vi "1DTurnMain.vi"() -> ()   [LabVIEW 2017]
panel:
  in  "StartAngle":dbl
  out "Done?":bool
  out "Vel":cluster{"Output":dbl, "dx/dt":dbl}(graph)={"Output"=0.0, "dx/dt"=-2.5707427177340247}
  in  "Gains":T1={"FFV"=0.0021, "FFA"=0.0001, "Vel PID"={"P"=0.002, "I"=0.0, "D"=0.0}} {"Vel PID"."D" format="%.3f"; "Vel PID"."I" format="%.3f"; "Vel PID"."P" format="%.3f"}
  out "Pos":dbl(graph)=90.04058722264358
  in  "Config":T2={"Gear Reduction"=15.0, "Wheel Radius (m)"=0.076, "# Motors"=6, "coeff of friction"=0.1, "Mass (kg)"=50.0, "Motor"={"Ke (V)"=0.0183, "R (ohms)"=0.09, "KT (Nm/A)"=0.0183, "Tf (Nm)"=0.4}}
  in  "TargetAngle":dbl=90.0
  in  "MaxVel":dbl=300.0
  in  "MaxAccel":dbl=400.0
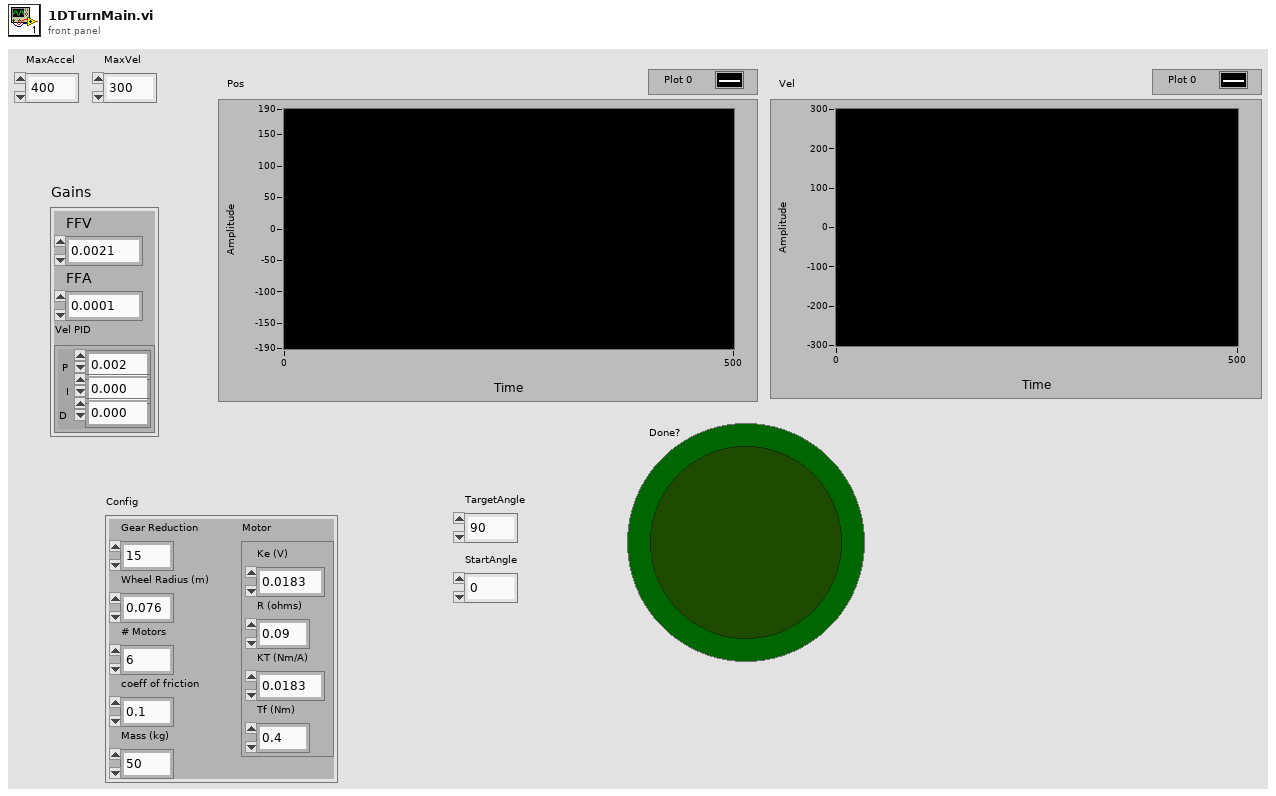
[diagram p1: front panel]
types:
  T1 = cluster{"FFV":dbl, "FFA":dbl, "Vel PID":cluster{"P":dbl, "I":dbl, "D":dbl}}
  T2 = cluster{"Gear Reduction":dbl, "Wheel Radius (m)":dbl, "# Motors":u32, "coeff of friction":dbl, "Mass (kg)":dbl, "Motor":cluster{"Ke (V)":dbl, "R (ohms)":dbl, "KT (Nm/A)":dbl, "Tf (Nm)":dbl}}
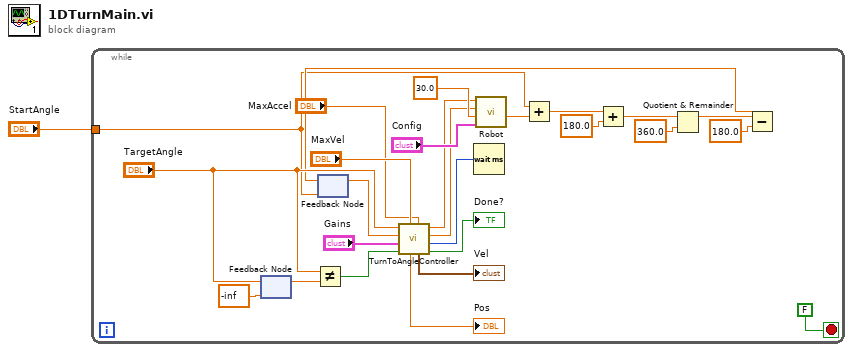
[diagram p0: block diagram]
diagram:
  n1 = while {
    tunnel: "StartAngle" -> [w2]
    stop <- FALSE stop-if-true
    n2 = feedback-in #1("TargetAngle") -> ()
    n3 = feedback #1(-inf ("TargetAngle")) -> (w13:dbl)
    n4 = Not Equal?(x="TargetAngle", y=w13) -> (x != y?=w12:bool)
    n5 = feedback #2(w2) -> (w18:dbl)
    n6 = call "TurnToAngleController.vi"("MaxAccel"="MaxAccel", "MaxVel"="MaxVel", "Reset"=w12, "Gains"="Gains", "CurrentAngle"=w18, "TargetAngle"="TargetAngle") -> ("Done"=→"Done?":bool, "Time Left"=w24:u32, "RightPower"=w19:dbl, "LeftPower"=w20:dbl, "VelGraph"=→"Vel":cluster{"Output":dbl, "dx/dt":dbl}, "Pos"=→"Pos":dbl)
    n7 = Wait (ms)(milliseconds to wait=w24) -> ()  [unwired: 1 out]
    n8 = call "Robot.vi"("Config"="Config", "WheelBase"=30.0, "Right Value"=w19, "Left Value"=w20) -> ("Angle"=w4:dbl)  [unwired: 5 in, 2 out]
    n9 = Add(x=w2, y=w4) -> (x+y=w3:dbl)
    n10 = Add(x=w3, y=180.0) -> (x+y=w9:dbl)
    n11 = Quotient & Remainder(x=w9, y=360.0) -> (x-y*floor(x/y)=w7:dbl)  [unwired: 1 out]
    n12 = Subtract(x=w7, y=180.0) -> (x-y=w5:dbl)
    n13 = feedback-in #2(w5) -> ()
  }
